vi "updateState.vi"(8 "error in (no error)":errorcluster, 10 "Monochromator in":refnum<class "Monochromator.lvclass">, 11 "MonoState in":refnum<class "MonoState.lvclass">) -> (0 "error out":errorcluster, 2 "Monochromator out":refnum<class "Monochromator.lvclass">, 3 "MonoState out":refnum<class "MonoState.lvclass">)   [LabVIEW 2016, in "MonoState.lvclass"]
uses:
  MonoState.lvclass
  Monochromator/Monochromator.lvclass
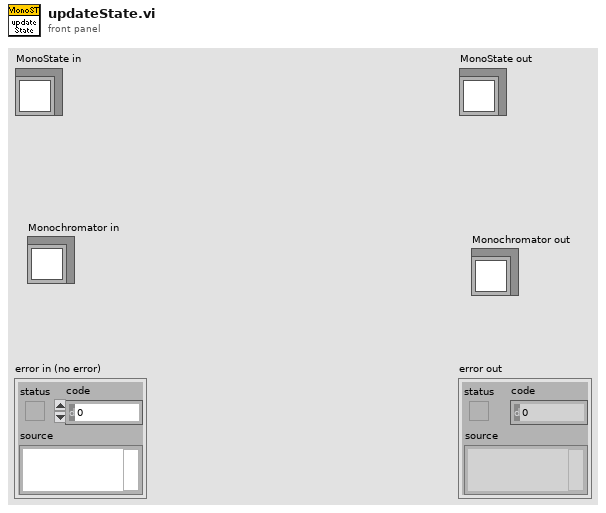
[diagram p1: front panel]
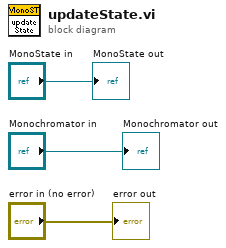
[diagram p0: block diagram]
diagram:
  "error out" <- "error in (no error)"
  "MonoState out" <- "MonoState in"
  "Monochromator out" <- "Monochromator in"
